vi "decomposeDataforGraph.vi"(11 "cluster":cluster{dbl, dbl, dbl, dbl, dbl, dbl}) -> (3 "Array":cluster{dbl[], dbl[]}[](array[cluster]))   [LabVIEW 2017]
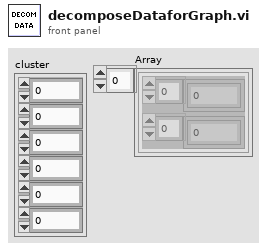
[diagram p1: front panel]
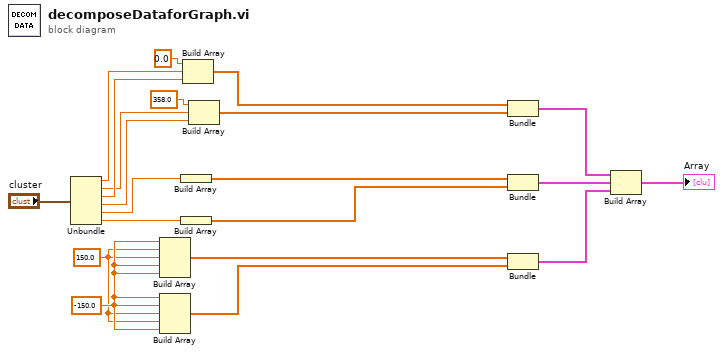
[diagram p0: block diagram]
diagram:
  w15 = -150.0
  w14 = 150.0
  n1 = Unbundle("cluster") -> (w4:dbl, w5:dbl, w19:dbl, w20:dbl, w17:dbl, w16:dbl)
  n2 = Build Array(w15, w14, w14, w15, w15) -> (w12:dbl[])
  n3 = Build Array(w15, w15, w14, w14, w15) -> (w13:dbl[])
  n4 = Build Array(w17) -> (w9:dbl[])
  n5 = Build Array(w16) -> (w10:dbl[])
  n6 = Build Array(0.0 ("element"), w4, w19) -> (w6:dbl[])
  n7 = Build Array(358.0 ("element"), w5, w20) -> (w7:dbl[])
  n8 = Bundle(w6, w7) -> (w8:cluster{dbl[], dbl[]})  [unwired: 1 in]
  n9 = Bundle(w9, w10) -> (w11:cluster{dbl[], dbl[]})  [unwired: 1 in]
  n10 = Bundle(w12, w13) -> (w18:cluster{dbl[], dbl[]})  [unwired: 1 in]
  n11 = Build Array(w8, w11, w18) -> (→"Array":cluster{dbl[], dbl[]}[])
